vi "Cont Acq Thermocouple Samples-Int Clk-Init.vi"(8 "error in":errorcluster, 10 "Rate":dbl=75.0 format="%0.2f", 11 "Physical Channel":tag="cDAQ1Mod1/ai1:15,cDAQ1Mod2/ai0:15,cDAQ1Mod3/ai0:15,cDAQ1Mod4/ai0:15") -> (0 "error out":errorcluster, 3 "Temp task out":refnum<k21>)   [LabVIEW 2009]
doc: "I. Description:\nThis example demonstrates how to make continuous, hardware-timed temperature measurement using a thermocouple.\n\nII. Instructions for Running:\n1. Specify the Physical Channel where you have connected the thermocouple.\n2. Enter the Minimum and Maximum temperature values in degrees C you expect to measure. A smaller range will allow a more accurate measurement.\n3. Enter the scan rate at which you want to run the acquisition.\n4. Specify the type of thermocouple you are using.\n5. Thermocouple measurements require cold-junction compensation (CJC) to correctly scale them. Specify the source of your cold-junction compensation.\n6. If your CJC source is \"Internal\", skip the rest of the steps.\n7. If your CJC source is \"Constant Value\", specify the value (usually room temperature) in degrees C.\n8. If your CJC source is \"Channel\", specify the CJC Channel name. \n9. Specify the appropriate Auto Zero Mode. See your device's hardware manual to find out if your device supports this attribute.\n\nIII. Block Diagram Steps:\n1. Create a Thermocouple (TC) temperature measurement channel.\n2. Get all the channels in the task.\n3. Convert channel(s) array to a comma-delimited channel string.\n4. This attribute is set to compensate for input offset errors. May not be supported by all devices*.\n5. Call the Timing VI to specify the hardware timing parameters. Use device's internal clock, continuous mode acquisition and the sample rate specified by the user.\n6. Call the Start VI to program and start the acquisition.\n7. Read N samples and plot it. By default, the Read VI reads all available samples, but you can specify how many samples to read at a time and the timeout value. Continue reading data until the stop button is pressed or an error occurs. \n8. Call the Clear Task VI to clear the Task.\n9. Use the popup dialog box to display an error if any.\n\n* If your device does not support Auto Zero Mode bypass Step 2, 3, and 4.\n\nIV. I/O Connections Overview:\nConnect your thermocouple to the terminals corresponding to the Physical Channel I/O Control value."
uses:
  <vilib>/DAQmx/configure/timing.llb/DAQmx Timing (Sample Clock).vi
  <vilib>/DAQmx/create/channels.llb/DAQmx Create Channel (AI-Temperature-Thermocouple).vi
  <vilib>/Utility/error.llb/DialogType.ctl
  <vilib>/DAQmx/read.llb/DAQmx Read (Analog 2D DBL NChan NSamp).vi
  Program Files/National Instruments/LabVIEW 2009/resource/objmgr/daqmx.rc
panel:
  out "size(s)":i32[](array[numeric])
  out "Array":dbl[](array[numeric])
  in  "number of samples per channel":i32=-1
  out "data":dbl[][](array[numeric]) format="%0.2f"
  out "Numeric":i32
  in  "stop":bool
  out "Measurement":dbl[][](graph)
  # "Timing Parameters"
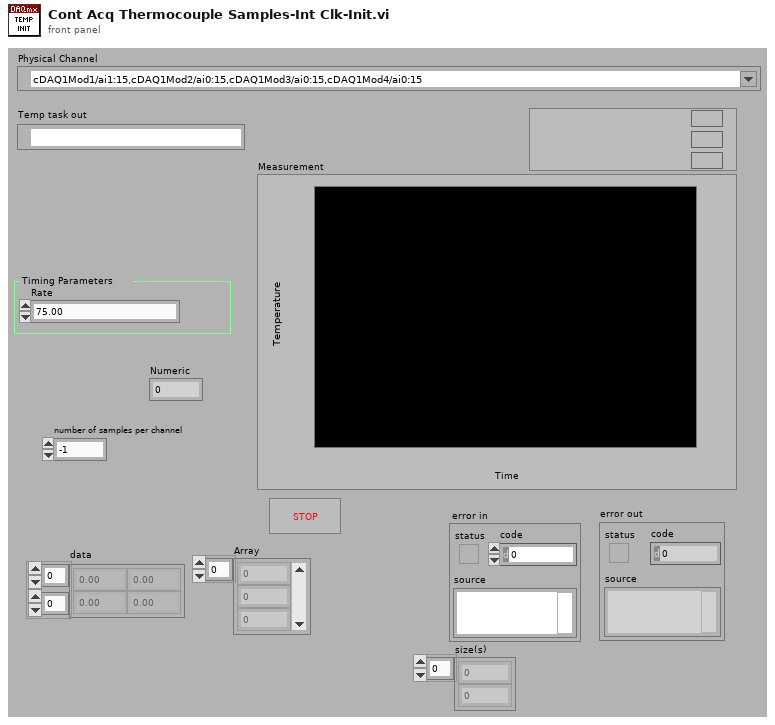
[diagram p1: front panel]
types:
  T1 = typedef "DialogType.ctl" = u16
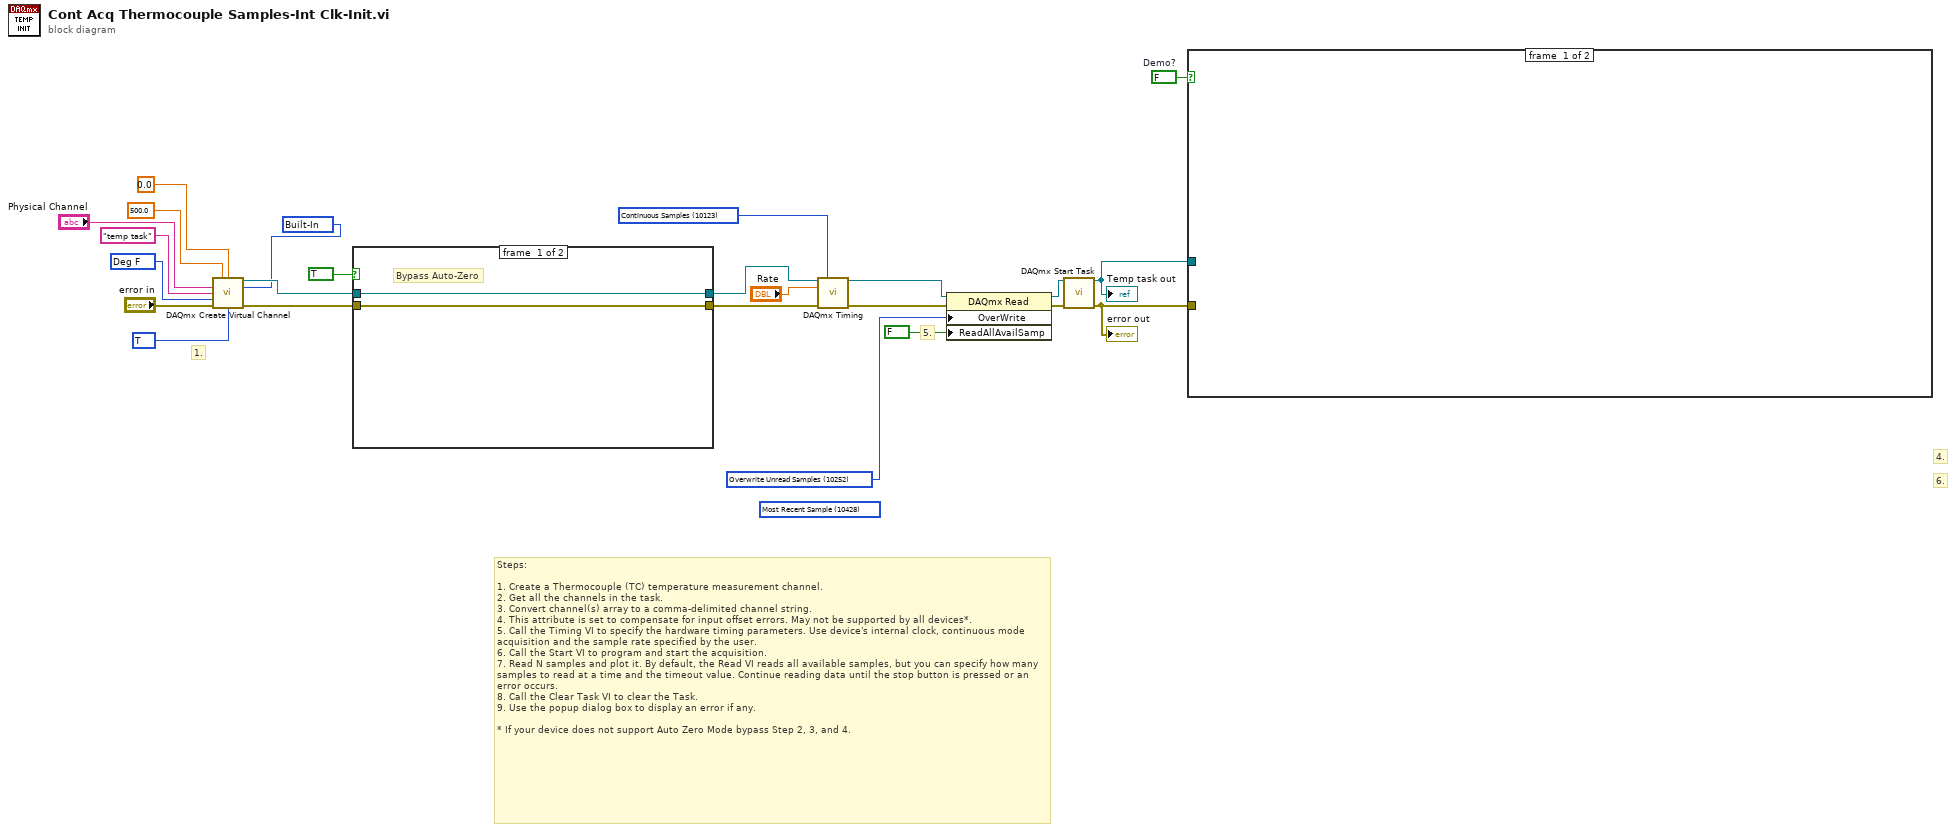
[diagram p0: block diagram]
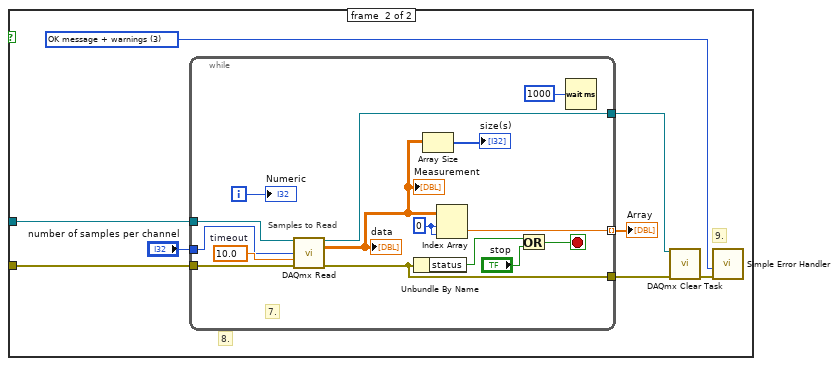
[diagram p2: hidden frame]
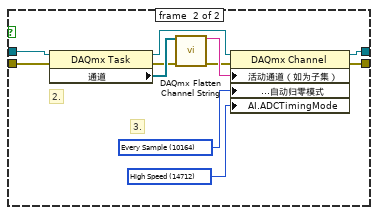
[diagram p3: hidden frame]
diagram:
  (unwired) 10428 items=["First Sample"=10424, "Current Read Position"=10425, "Reference Trigger"=10426, "First Pretrigger Sample"=10427, "Most Recent Sample"=10428] ("RelativeTo")
  w7 = 10252 items=["Overwrite Unread Samples"=10252, "Do Not Overwrite Unread Samples"=10159] ("OverWrite")
  w10 = FALSE  # Demo?
  w11 = 10144 items=["Deg C"=10143, "Deg F"=10144, "Kelvins"=10325, "Deg R"=10145, "From Custom Scale"=10065] ("units")
  w20 = 10086 items=["J"=10072, "K"=10073, "N"=10077, "R"=10082, "S"=10085, "T"=10086, "B"=10047, "E"=10055] ("Thermocouple Type")
  w12 = 10200 items=["Built-In"=10200, "Constant Value"=10116, "Channel"=10113] ("CJC Source")
  w17 = 10123 items=["Finite Samples"=10178, "Continuous Samples"=10123] ("sample mode")
  # "4."
  # "5."
  # "6."
  # "1."
  # "Steps: \n\n1. Create a Thermocouple (TC) temperature measurement channel.\n2. Get all the channels in the task.\n3. Convert channel(s) array to a comma-delimited channel string.\n4. This attribute is set to compensate for input offset errors. May not be supported by all devices*.\n5. Call the Timing VI to specify the hardware timing parameters. Use device's internal clock, continuous mode acquisition and the sample rate specified by the user.\n6. Call the Start VI to program and start the acquisition.\n7. Read N samples and plot it. By default, the Read VI reads all available samples, but you can specify how many samples to read at a time and the timeout value. Continue reading data until the stop button is pressed or an error occurs. \n8. Call the Clear Task VI to clear the Task.\n9. Use the popup dialog box to display an error if any.\n\n* If your device does not support Auto Zero Mode bypass Step 2, 3, and 4."
  n1 = call-poly <vilib>:"DAQmx Create Virtual Channel.vi"("maximum value"=500.0 ("Maximum Value (deg C)"), "minimum value"=0.0 ("Minimum Value (degF)"), "physical channels"="Physical Channel", "cjc source"=w12, "name to assign"="temp task", "units"=w11, "error in"="error in", "thermocouple type"=w20) -> ("task out"=w19:refnum<k21>, "error out"=w18:errorcluster)  [unwired: 6 in]
  n2 = case shown="True" TRUE ("SCXI Module?") {
    tunnel: w19 -> [w25 w36]
    tunnel: w18 -> [w26 w35]
    tunnel: [w25 w31] -> w16
    tunnel: [w26 w30] -> w15
    frame #0 {
      # "Bypass Auto-Zero"
    }
    frame #1 {
      w27 = 14712 items=["High Resolution"=10195, "High Speed"=14712, "Best 50 Hz Rejection"=14713, "Best 60 Hz Rejection"=14714, "Custom"=10137] ("AI.ADCTimingMode")
      w37 = 10164 items=["None"=10230, "Once"=10244, "Every Sample"=10164] ("Auto Zero Mode")
      # "3."
      # "2."
      n3 = property class="DAQmx Task"(reference=w36, error in=w35) -> (reference out=w34:refnum<k21>, error out=w29:errorcluster, "通道"=w33:refnum<k21>[])
      n4 = call <vilib>:"DAQmx Flatten Channel String.vi"("names in"=w33, "error in"=w29) -> ("names out"=w32:string, "error out"=w28:errorcluster)  [unwired: 12 in]
      n5 = property class="DAQmx Channel"(reference=w34, error in=w28, "活动通道（如为子集）"=w32, "模拟输入:常规属性:高级:高精度设置:自动归零模式"=w37, "AI.ADCTimingMode"=w27) -> (reference out=w31:refnum<k21>, error out=w30:errorcluster)
    }
  }
  n6 = call-poly <vilib>:"DAQmx Timing.vi"("task/channels in"=w16, "sample mode"=w17, "rate"="Rate", "error in"=w15) -> ("task out"=w8:refnum<k21>, "error out"=w6:errorcluster)  [unwired: 10 in]
  n7 = property class="DAQmx Read"(reference=w8, error in=w6, "OverWrite"=w7, "ReadAllAvailSamp"=FALSE) -> (reference out=w5:refnum<k21>, error out=w4:errorcluster)
  n8 = call <vilib>:"DAQmx Start Task.vi"("task/channels in"=w5, "error in"=w4) -> ("task out"=w23:refnum<k21>, "error out"=w24:errorcluster)  [unwired: 12 in]
  "Temp task out" <- w23
  "error out" <- w24
  n9 = case shown="False" w10 {
    tunnel: w24 -> [_ w43]
    tunnel: w23 -> [_ w42]
    frame #0 {
    }
    frame #1 {
      w40 = T1 3 items=["no dialog", "OK message", "continue or stop message", "OK message + warnings", "continue/stop + warnings"] ("type of dialog (OK msg:1)")
      # "9."
      # "8."
      n10 = while {
        tunnel: [w57] -> w44
        tunnel: w42 -> [w60]
        tunnel: w43 -> [w59]
        tunnel: [w58] -> w41
        tunnel: "number of samples per channel" -> [w52]
        tunnel: [w49] -> w38 mode=indexing
        i -> [w51]
        stop <- w55 stop-if-true
        w50 = 0 ("index (row)")
        w53 = 10.0  # timeout
        # "Samples to Read"
        # "7."
        n11 = call-poly <vilib>:"DAQmx Read.vi"("task/channels in"=w60, "number of samples per channel"=w52, "timeout"=w53, "error in"=w59) -> ("task out"=w58:refnum<k21>, "data"=w48:dbl[][], "error out"=w57:errorcluster)  [unwired: 9 in]
        "Measurement" <- w48
        "data" <- w48
        n12 = Unbundle By Name(w57) -> ("status"=w56:bool)
        n13 = Array Size(array=w48) -> (size(s)=→"size(s)":i32[])
        n14 = Index Array(array=w48, index (row)=w50, index (col)=w50) -> (element=w49:dbl)
        n15 = Or(x=w56, y="stop") -> (x .or. y?=w55:bool)
        n16 = Wait (ms)(milliseconds to wait=u32 1000) -> ()  [unwired: 1 out]
        "Numeric" <- w51
      }
      "Array" <- w38
      n17 = call <vilib>:"DAQmx Clear Task.vi"("task in"=w41, "error in"=w44) -> ("error out"=w45:errorcluster)  [unwired: 13 in]
      n18 = call <vilib>:"Simple Error Handler.vi"("type of dialog (OK msg:1)"=w40, "error in (no error)"=w45) -> ()  [unwired: 3 in, 5 out]
    }
  }
